vi "corrected_turn_rate.vi"(9 "Time between reading":dbl=0.125, 10 "Previous Heading":dbl, 11 "Current Heading":dbl) -> (1 "difference":dbl, 2 "Previous Heading":dbl, 3 "Turn rate":dbl)   [LabVIEW 2009]
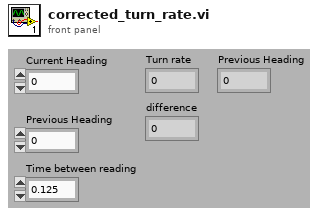
[diagram p1: front panel]
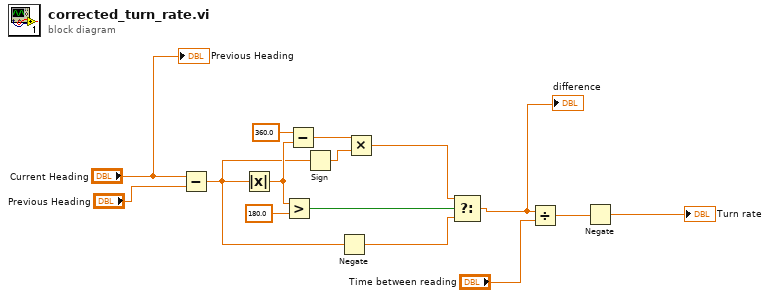
[diagram p0: block diagram]
diagram:
  n1 = Subtract(x="Current Heading", y="Previous Heading") -> (x-y=w4:dbl)
  n2 = Absolute Value(x=w4) -> (abs(x)=w6:dbl)
  n3 = Greater?(x=w6, y=180.0) -> (0:w11:bool)
  n4 = Subtract(x=360.0, y=w6) -> (x-y=w9:dbl)
  n5 = Sign(1:w4) -> (0:w8:dbl)
  n6 = Negate(x=w4) -> (-x=w5:dbl)
  n7 = Multiply(x=w9, y=w8) -> (x*y=w7:dbl)
  n8 = Select(t=w7, s=w11, f=w5) -> (s? t:f=w3:dbl)
  "difference" <- w3
  n9 = Divide(x=w3, y="Time between reading") -> (x/y=w2:dbl)
  n10 = Negate(x=w2) -> (-x=→"Turn rate":dbl)
  "Previous Heading" <- "Current Heading"
